vi "SetDefaultModeValue.vi"(1 "Array in":T1[](array[typedef]), 2 "index":i32, 3 "Amplititute":dbl) -> (0 "output array":T1[](array[typedef]))   [LabVIEW 2018]
uses:
  Controls/Holo Setting.ctl
  Controls/Buttons/Running Button.ctl
  Controls/Zernike Polynominals.ctl
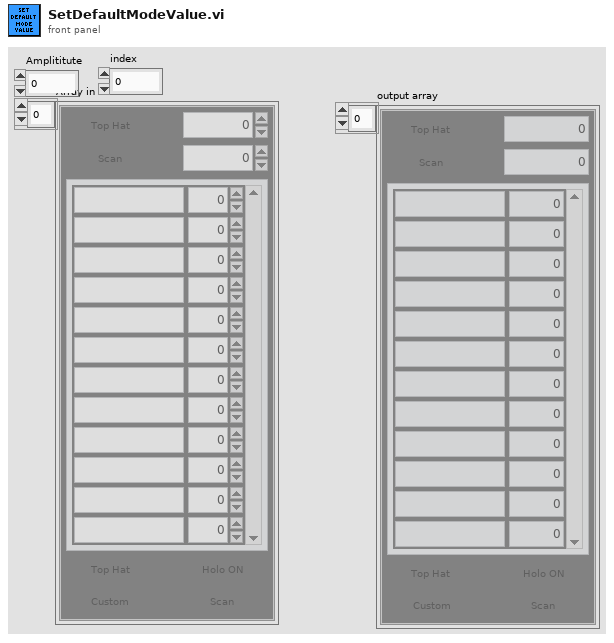
[diagram p1: front panel]
types:
  T1 = typedef "Holo Setting.ctl" = cluster{"Holo On":T2, "Scan":T2, "X":i16, "Y":i16, "Zernike Polynominals":T3, "Top Hat":T2, "Vortex":T2, "Clockwise":T2, "Custom":T2}
  T2 = typedef "Running Button.ctl" = bool
  T3 = typedef "Zernike Polynominals.ctl" = cluster{"Aberration Name":string, "Numeric":dbl}[]
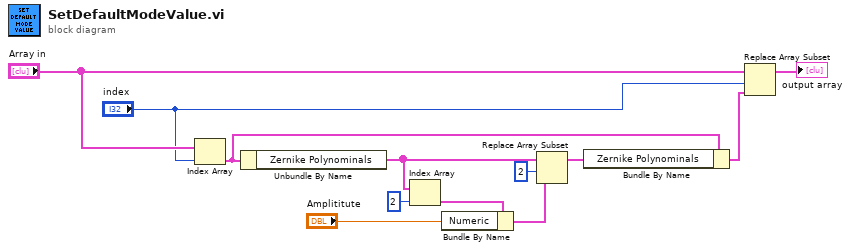
[diagram p0: block diagram]
diagram:
  n1 = Index Array(array="Array in", index="index") -> (element=w10:T1)
  n2 = Unbundle By Name(w10) -> ("Zernike Polynominals"=w6:T3)
  n3 = Index Array(array=w6, index=2) -> (element=w4:cluster{"Aberration Name":string, "Numeric":dbl})
  n4 = Bundle By Name(cluster=w4, "Numeric"="Amplititute") -> (w8:cluster{"Aberration Name":string, "Numeric":dbl})
  n5 = Replace Array Subset(array=w6, new element=w8, index=2) -> (w11:T3)
  n6 = Bundle By Name(cluster=w10, "Zernike Polynominals"=w11) -> (w12:T1)
  n7 = Replace Array Subset(array="Array in", new element=w12, index="index") -> (→"output array":T1[])
